vi "Do.vi"(8 "error in (no error)":errorcluster caption="错误输入（无错误）", 10 "Actor in":refnum<class "Actor.lvclass"> caption="操作者输入", 11 "编译图形消息":refnum<class "编译图形消息.lvclass">) -> (0 "error out":errorcluster caption="错误输出", 2 "Actor out":refnum<class "Actor.lvclass"> caption="操作者输出")   [LabVIEW 2018, in "程序响应.lvlib" / "编译图形消息.lvclass"]
doc: "本VI通过对操作者调用合适的方法，将消息发送给操作者。"
uses:
  <vilib>/ActorFramework/Actor/Actor.lvclass
  C:/Program Files (x86)/National Instruments/LabVIEW 2018/vi.lib/ActorFramework/Actor/Actor.lvclass
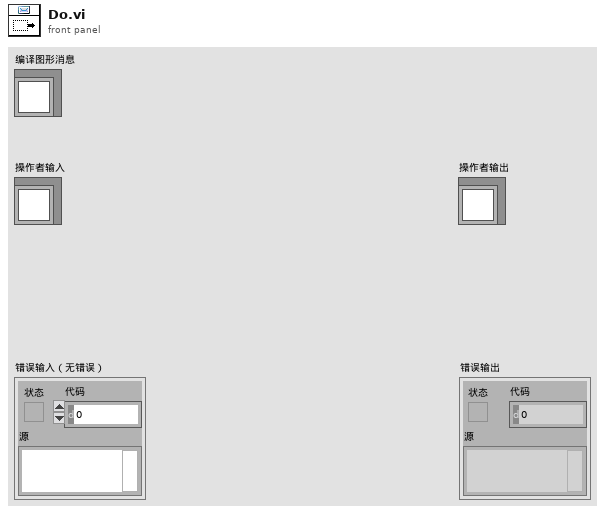
[diagram p1: front panel]
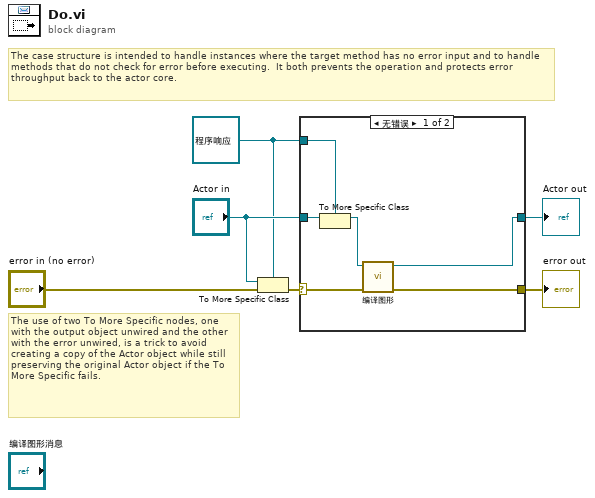
[diagram p0: block diagram]
diagram:
  w1 = refnum<class "程序响应.lvclass"> refnum ("Actor in")
  # "The use of two To More Specific nodes, one with the output object unwired and the other with the error unwired, is a trick to avoid creating a copy of the Actor object while still preserving the original Actor object if the To More Specific fails."
  # "The case structure is intended to handle instances where the target method has no error input and to handle methods that do not check for error before executing.  It both prevents the operation and protects error throughput back to the actor core."
  n1 = To More Specific Class(target class=w1, reference="Actor in", error in="error in (no error)") -> (error out=w5:errorcluster)  [unwired: 1 out]
  n2 = case shown="无错误" w5 {
    selector: w5 -> [w10 w14]
    tunnel: [w12 w14] -> w4
    tunnel: [w11 w13] -> w3
    tunnel: "Actor in" -> [w9 w13]
    tunnel: w1 -> [w8 _]
    frame No Error {
      n3 = To More Specific Class(target class=w8, reference=w9) -> (specific class reference=w7:refnum<class "程序响应.lvclass">)  [unwired: 1 in, 1 out]
      n4 = call-dynamic "编译图形.vi"("error in (no error)"=w10, "程序响应 输入"=w7) -> ("error out"=w12:errorcluster, "程序响应 输出"=w11:refnum<class "程序响应.lvclass">)  [unwired: 8 in]
    }
    frame Error {
      # "If type check fails, pass the original object out again."
    }
  }
  "error out" <- w4
  "Actor out" <- w3
